vi "HEWH MCp_DeltaT.vi"(0 "Mass of water All (lbm)":dbl[](array[numeric]), 5 "CpHW (BTU/(lbm °F))":dbl[](array[numeric]), 9 "T del_all - Outlet Temps (°F)":dbl[](array[numeric]), 11 "error in (no error)":errorcluster, 12 "T in_all - Inlet Temps (°F)":dbl[](array[numeric]), 14 "nu_r":dbl) -> (4 "QHW":dbl, 15 "error out":errorcluster)   [LabVIEW 2023]
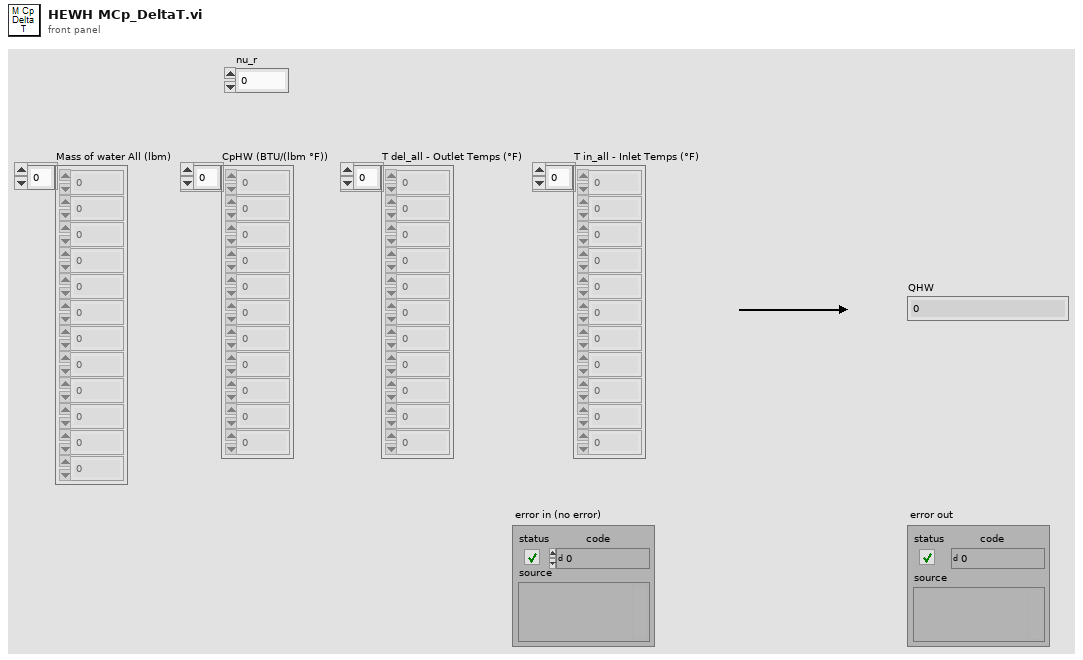
[diagram p1: front panel]
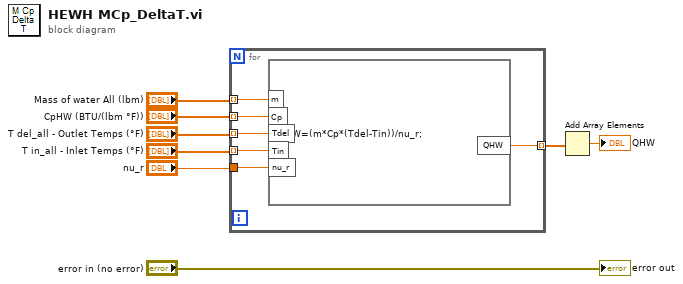
[diagram p0: block diagram]
diagram:
  n1 = for {
    tunnel: "Mass of water All (lbm)" -> [w14] mode=indexing
    tunnel: "CpHW (BTU/(lbm °F))" -> [w13] mode=indexing
    tunnel: "T del_all - Outlet Temps (°F)" -> [w12] mode=indexing
    tunnel: "T in_all - Inlet Temps (°F)" -> [w11] mode=indexing
    tunnel: "nu_r" -> [w10]
    tunnel: [w9] -> w2 mode=indexing
    n2 = formula code="QHW=(m*Cp*(Tdel-Tin))/nu_r;"("m"=w14, "Cp"=w13, "Tdel"=w12, "Tin"=w11, "nu_r"=w10) -> ("QHW"=w9:dbl)
  }
  n3 = Add Array Elements(numeric array=w2) -> (sum=→"QHW":dbl)
  "error out" <- "error in (no error)"
